vi "Write AO Channels.vi"(8 "error in (no error)":errorcluster, 10 "AO Channels":T1 {"Frequency" format="%.3g"; "Offset" min=0.0001 max=10000.0 format="%.3g"; "Amplitude" format="%5.2p"; "Channel" min=0 max=10 format="%5.2p"}, 11 "Generator in":refnum<class "Generator.lvclass">) -> (0 "error out":errorcluster, 3 "Generator out":refnum<class "Generator.lvclass">)   [LabVIEW 2019, in "Generator.lvclass"]
uses:
  Generator.lvclass
  typedefs/AO.Channel--Cluster--Array.ctl
  typedefs/AO.Channel--Cluster.ctl
  typedefs/AO.Channel.Function--Enum.ctl
  Generator.lvclass/Generator.ctl
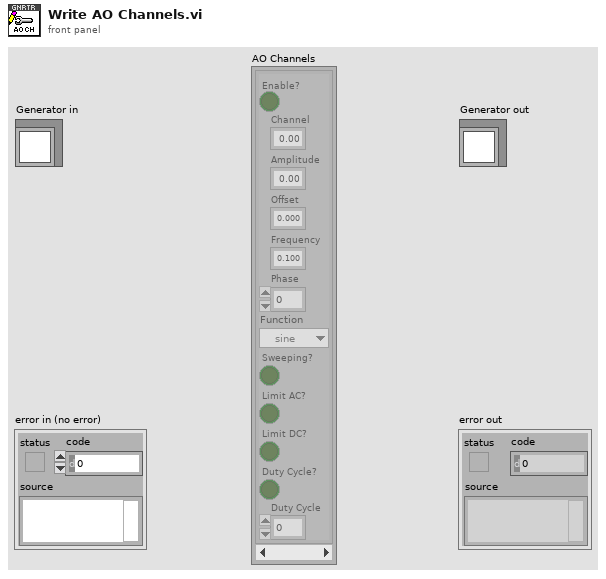
[diagram p1: front panel]
types:
  T1 = typedef "Generator.lvclass/AO.Channel--Cluster--Array.ctl" = T2[]
  T2 = typedef "Generator.lvclass/AO.Channel--Cluster.ctl" = cluster{"Enable?":bool, "Channel":i32, "Amplitude":dbl, "Offset":dbl, "Frequency":dbl, "Phase":dbl, "Function":T3, "Sweeping?":bool, "Limit AC?":bool, "Limit DC?":bool, "Duty Cycle?":bool, "Duty Cycle":dbl}
  T3 = typedef "Generator.lvclass/AO.Channel.Function--Enum.ctl" = enum16{"sine", "square", "triangle", "saw"}
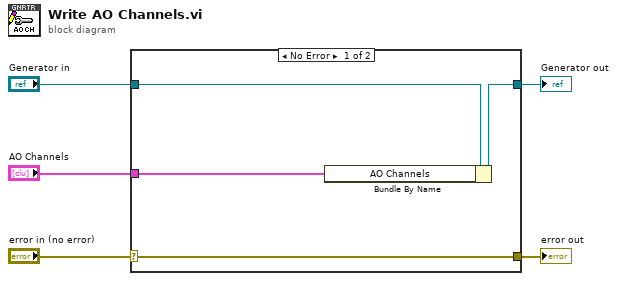
[diagram p0: block diagram]
diagram:
  n1 = case shown="No Error" "error in (no error)" {
    selector: "error in (no error)" -> [w9 w10]
    tunnel: [w9 w10] -> w4
    tunnel: [w7 w11] -> w2
    tunnel: "Generator in" -> [w8 w11]
    tunnel: "AO Channels" -> [w6 _]
    frame No Error {
      n2 = Bundle By Name(cluster=w8, "AO Channels"=w6) -> (w7:refnum<class "Generator.lvclass">)
    }
    frame Error {
    }
  }
  "error out" <- w4
  "Generator out" <- w2
